vi "Autonomous Independent.vi"   [LabVIEW 2015]
doc: "This VI is called when autonomous begins, and will automatically be terminated when autonomous ends. You can carry out timed or sensor driven robot movement independently without needing to return to the caller."
uses:
  <vilib>/Rock Robotics/WPI/Relay/WPI_RelayValue.ctl
panel:
  # "Be sure to right-click and choose Data Operations>>Make Current Value default if you want to save the array values with the VI"
types:
  T1 = typedef "WPI_RelayDevRef.ctl" = cluster{"DevStatus":errorcluster, "Relay Channel":T2, "Relay Direction":T3}
  T2 = typedef "FPGA_DIORelayChannel.ctl" = enum8{"Relay 0", "Relay 1", "Relay 2", "Relay 3", "Invalid"}
  T3 = typedef "WPI_RelayDirection.ctl" = enum16{"Both directions", "Forward only", "Reverse only"}
  T4 = typedef "WPI_MotorControlDeviceRef.ctl" = cluster{"DeviceStatus":errorcluster, "Type":T5, "PWM":cluster{"PWM Channel":T6, "DeadBand":T7}, "CAN":cluster{"Device Number":u8, "Control Mode":T8, "Semaphore":T9, "Max Vout":dbl, "TalonSRX Control Mode":T10}, "Invert":bool}
  T5 = typedef "WPI_MotorControlType.ctl" = enum16{"PWM", "CAN", "CANTalonSRX"}
  T6 = typedef "FPGA_DIOPWMChannel.ctl" = enum8{"PWM 0", "PWM 1", "PWM 2", "PWM 3", "PWM 4", "PWM 5", "PWM 6", "PWM 7", "PWM 8", "PWM 9", "PWM MXP 0", "PWM MXP 1", "PWM MXP 2", "PWM MXP 3", "PWM MXP 4", "PWM MXP 5", "PWM MXP 6", "PWM MXP 7", "PWM MXP 8", "PWM MXP 9", "Invalid"}
  T7 = typedef "WPI_PWMDeadband.ctl" = cluster{"Name":string, "maxPositivePwm":i32, "minPositivePwm":i32, "centerPwm":i32, "maxNegativePwm":i32, "minNegativePwm":i32, "angularRange":u16}
  T8 = typedef "WPI_CANJaguar_ControlMode.ctl" = enum8{"Percent VBus", "Current", "Speed", "Position", "Voltage"}
  T9 = typedef "Semaphore RefNum" = refnum<k1>
  T10 = typedef "WPI_CANTalonSRX_APIControlMode.ctl" = enum8{"Percent VBus", "Speed", "Position", "Slave", "Unchanged / Invalid", "Voltage Compensation", "Current", "Motion Profile"}
  T11 = typedef "WPI_RelayValue.ctl" = enum16{"Off", "On", "Forward", "Reverse"}
  T12 = typedef "WPI_SwitchDevRef.ctl" = cluster{"DevStatus":errorcluster, "DIO Channel":T13, "CntIndex":T14, "Normally Closed":bool}
  T13 = typedef "FPGA_DIOChannel.ctl" = enum8{"DIO 0", "DIO 1", "DIO 2", "DIO 3", "DIO 4", "DIO 5", "DIO 6", "DIO 7", "DIO 8", "DIO 9", "DIO MXP 0", "DIO MXP 1", "DIO MXP 2", "DIO MXP 3", "DIO MXP 4", "DIO MXP 5", "DIO MXP 6", "DIO MXP 7", "DIO MXP 8", "DIO MXP 9", "DIO MXP 10", "DIO MXP 11", "DIO MXP 12", "DIO MXP 13", "DIO MXP 14", "DIO MXP 15", "Invalid"}
  T14 = typedef "FPGA_CounterCtrSystemIndex.ctl" = enum8{"Ctr 0", "Ctr 1", "Ctr 2", "Ctr 3", "Ctr 4", "Ctr 5", "Ctr 6", "Ctr 7", "Invalid"}
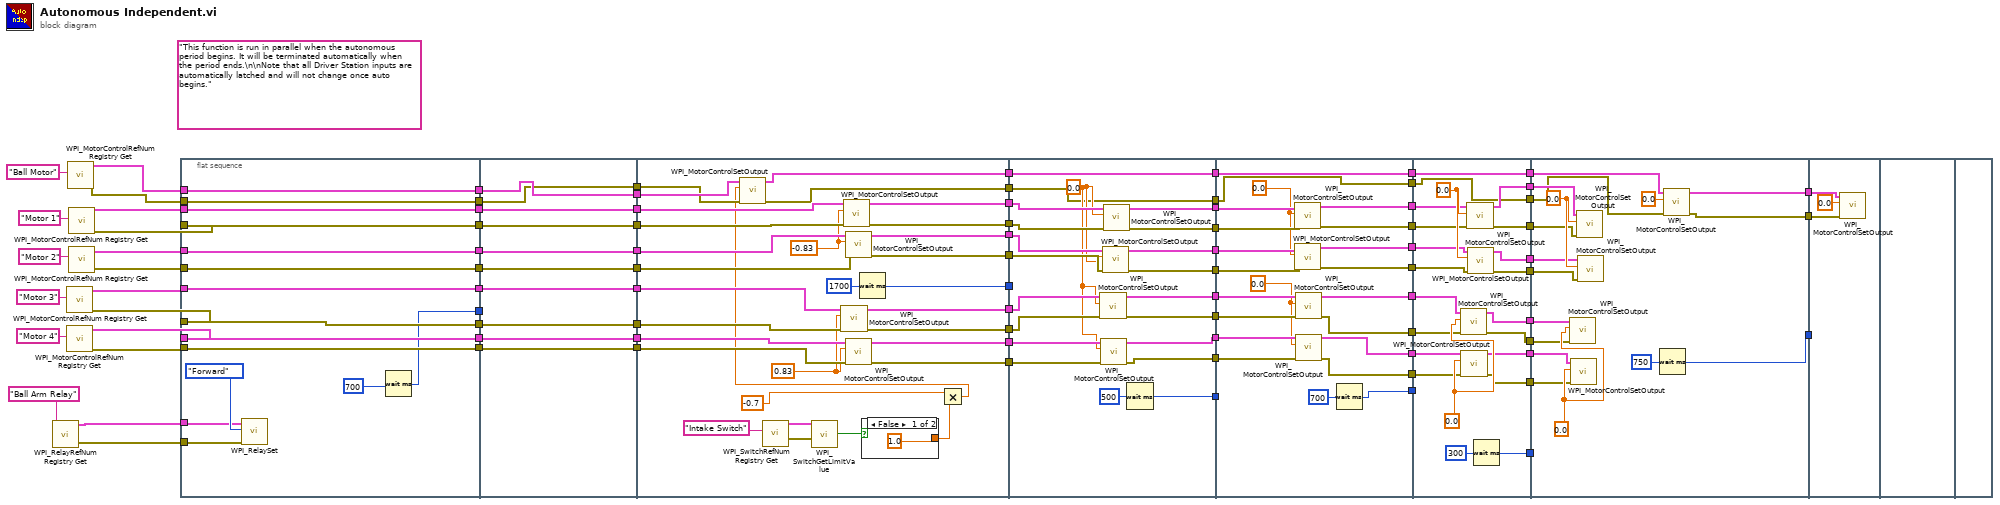
[diagram p0: block diagram]
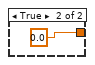
[diagram p2: hidden frame]
diagram:
  (unwired) "This function is run in parallel when the autonomous period begins. It will be terminated automatically when the period ends.\n\nNote that all Driver Station inputs are automatically latched and will not change once auto begins."
  n1 = call <vilib>:"WPI_RelayRefNum Registry Get.vi"("refnum name"="Ball Arm Relay") -> ("error out"=w72:errorcluster, "RelayDevRef"=w73:T1)  [unwired: 9 in]
  n2 = call <vilib>:"WPI_MotorControlRefNum Registry Get.vi"("refnum name"="Motor 3") -> ("error out"=w80:errorcluster, "MotorControlDevRef"=w79:T4)  [unwired: 9 in]
  n3 = call <vilib>:"WPI_MotorControlRefNum Registry Get.vi"("refnum name"="Motor 4") -> ("error out"=w81:errorcluster, "MotorControlDevRef"=w82:T4)  [unwired: 9 in]
  n4 = call <vilib>:"WPI_MotorControlRefNum Registry Get.vi"("refnum name"="Ball Motor") -> ("error out"=w51:errorcluster, "MotorControlDevRef"=w52:T4)  [unwired: 9 in]
  n5 = call <vilib>:"WPI_MotorControlRefNum Registry Get.vi"("refnum name"="Motor 1") -> ("error out"=w76:errorcluster, "MotorControlDevRef"=w75:T4)  [unwired: 9 in]
  n6 = call <vilib>:"WPI_MotorControlRefNum Registry Get.vi"("refnum name"="Motor 2") -> ("error out"=w78:errorcluster, "MotorControlDevRef"=w77:T4)  [unwired: 9 in]
  n7 = flat-sequence {
    tunnel: w75 -> [w94]
    tunnel: w76 -> [w95]
    tunnel: w77 -> [w96]
    tunnel: w78 -> [w97]
    tunnel: w79 -> [w98]
    tunnel: w80 -> [w99]
    tunnel: w81 -> [w100]
    tunnel: w82 -> [w101]
    tunnel: [w101] -> w70
    tunnel: [w100] -> w68
    tunnel: [w99] -> w66
    tunnel: [w98] -> w64
    tunnel: [w97] -> w62
    tunnel: [w96] -> w60
    tunnel: [w95] -> w58
    tunnel: [w94] -> w56
    tunnel: w73 -> [w92]
    tunnel: w72 -> [w91]
    tunnel: [w89] -> w54
    tunnel: [w88] -> w53
    tunnel: w52 -> [w88]
    tunnel: w51 -> [w87]
    tunnel: [w87] -> w50
    tunnel: w70 -> [w111]
    tunnel: [w111] -> w69
    tunnel: w68 -> [w110]
    tunnel: [w110] -> w67
    tunnel: w66 -> [w109]
    tunnel: [w109] -> w65
    tunnel: w64 -> [w108]
    tunnel: [w108] -> w63
    tunnel: w62 -> [w107]
    tunnel: [w107] -> w61
    tunnel: w60 -> [w106]
    tunnel: [w106] -> w59
    tunnel: w58 -> [w105]
    tunnel: [w105] -> w57
    tunnel: w56 -> [w104]
    tunnel: [w104] -> w55
    tunnel: w54 -> [_]
    tunnel: w53 -> [w103]
    tunnel: w50 -> [w102]
    tunnel: [w103] -> w49
    tunnel: [w102] -> w48
    tunnel: [w132] -> w47
    tunnel: [w131] -> w46
    tunnel: [w130] -> w45
    tunnel: [w129] -> w44
    tunnel: [w128] -> w43
    tunnel: [w127] -> w42
    tunnel: [w126] -> w41
    tunnel: [w125] -> w40
    tunnel: w69 -> [w142]
    tunnel: w67 -> [w141]
    tunnel: w65 -> [w140]
    tunnel: w63 -> [w139]
    tunnel: w61 -> [w138]
    tunnel: w59 -> [w137]
    tunnel: w57 -> [w136]
    tunnel: w55 -> [w135]
    tunnel: [w123] -> w39
    tunnel: w49 -> [w122]
    tunnel: w48 -> [w121]
    tunnel: [w113] -> w9
    tunnel: [w112] -> w6
    tunnel: w47 -> [w158]
    tunnel: w46 -> [w159]
    tunnel: w45 -> [w160]
    tunnel: w44 -> [w161]
    tunnel: w43 -> [w163]
    tunnel: w42 -> [w162]
    tunnel: w41 -> [w165]
    tunnel: w40 -> [w164]
    tunnel: w39 -> [_]
    tunnel: [w156] -> w38
    tunnel: [w155] -> w37
    tunnel: [w154] -> w36
    tunnel: [w153] -> w35
    tunnel: [w152] -> w34
    tunnel: [w151] -> w33
    tunnel: [w150] -> w32
    tunnel: [w149] -> w31
    tunnel: [w148] -> w30
    tunnel: [w146] -> w10
    tunnel: w9 -> [w146]
    tunnel: [w145] -> w7
    tunnel: w6 -> [w145]
    tunnel: w38 -> [w187]
    tunnel: w37 -> [w186]
    tunnel: w36 -> [w185]
    tunnel: w35 -> [w184]
    tunnel: w34 -> [w183]
    tunnel: w33 -> [w182]
    tunnel: w32 -> [w181]
    tunnel: w31 -> [w180]
    tunnel: [w178] -> w29
    tunnel: w30 -> [_]
    tunnel: [w176] -> w28
    tunnel: [w175] -> w27
    tunnel: [w174] -> w26
    tunnel: [w173] -> w25
    tunnel: [w172] -> w24
    tunnel: [w171] -> w23
    tunnel: [w170] -> w22
    tunnel: [w169] -> w21
    tunnel: [w168] -> w11
    tunnel: w10 -> [w168]
    tunnel: [w167] -> w8
    tunnel: w7 -> [w167]
    tunnel: w29 -> [_]
    tunnel: w28 -> [w207]
    tunnel: w27 -> [w206]
    tunnel: w26 -> [w205]
    tunnel: w25 -> [w204]
    tunnel: w24 -> [w203]
    tunnel: w23 -> [w202]
    tunnel: w22 -> [w201]
    tunnel: w21 -> [w200]
    tunnel: [w199] -> w20
    tunnel: [w197] -> w19
    tunnel: [w196] -> w18
    tunnel: [w195] -> w17
    tunnel: [w194] -> w16
    tunnel: [w193] -> w15
    tunnel: [w192] -> w14
    tunnel: [w191] -> w13
    tunnel: [w190] -> w12
    tunnel: w11 -> [w189]
    tunnel: w8 -> [w188]
    tunnel: [w189] -> w5
    tunnel: [w188] -> w4
    tunnel: w20 -> [_]
    tunnel: w19 -> [w224]
    tunnel: w18 -> [w223]
    tunnel: w17 -> [w222]
    tunnel: w16 -> [w221]
    tunnel: w15 -> [w220]
    tunnel: w14 -> [w219]
    tunnel: w13 -> [w218]
    tunnel: w12 -> [w217]
    tunnel: w5 -> [w216]
    tunnel: w4 -> [w215]
    tunnel: [w212] -> w3
    tunnel: [w211] -> w2
    tunnel: [w210] -> w1
    tunnel: w3 -> [_]
    tunnel: w2 -> [w229]
    tunnel: w1 -> [w228]
    frame #0 {
      n8 = call <vilib>:"WPI_RelaySet.vi"("error in (no error)"=w91, "RelayValue"=WPI_RelayValue."Forward", "RelayDevRef"=w92) -> ()  [unwired: 7 in, 2 out]
      n9 = Wait (ms)(milliseconds to wait=u32 700) -> (millisecond timer value=w89:u32)
    }
    frame #1 {
    }
    frame #2 {
      w133 = 0.83
      w134 = -0.83
      n10 = call <vilib>:"WPI_SwitchRefNum Registry Get.vi"("refnum name"="Intake Switch") -> ("error out"=w119:errorcluster, "SwitchDevRef"=w120:T12)  [unwired: 9 in]
      n11 = call <vilib>:"WPI_SwitchGetLimitValue.vi"("error in (no error)"=w119, "SwitchDevRef"=w120) -> ("Switch Pressed"=w114:bool)  [unwired: 7 in, 2 out]
      n12 = call <vilib>:"WPI_MotorControlSetOutput.vi"("error in (no error)"=w140, "Output"=w133, "MotorControlDevRef"=w139) -> ("error out"=w127:errorcluster, "MotorControlDevRef"=w128:T4)  [unwired: 6 in, 1 out]
      n13 = call <vilib>:"WPI_MotorControlSetOutput.vi"("error in (no error)"=w136, "Output"=w134, "MotorControlDevRef"=w135) -> ("error out"=w131:errorcluster, "MotorControlDevRef"=w132:T4)  [unwired: 6 in, 1 out]
      n14 = call <vilib>:"WPI_MotorControlSetOutput.vi"("error in (no error)"=w138, "Output"=w134, "MotorControlDevRef"=w137) -> ("error out"=w129:errorcluster, "MotorControlDevRef"=w130:T4)  [unwired: 6 in, 1 out]
      n15 = call <vilib>:"WPI_MotorControlSetOutput.vi"("error in (no error)"=w141, "Output"=w133, "MotorControlDevRef"=w142) -> ("error out"=w125:errorcluster, "MotorControlDevRef"=w126:T4)  [unwired: 6 in, 1 out]
      n16 = Wait (ms)(milliseconds to wait=u32 1700) -> (millisecond timer value=w123:u32)
      n17 = case shown="False" w114 {
        tunnel: [1.0 0.0] -> w117
        frame False {
        }
        frame True {
        }
      }
      n18 = Multiply(x=-0.7 ("Output"), y=w117) -> (x*y=w115:dbl)
      n19 = call <vilib>:"WPI_MotorControlSetOutput.vi"("error in (no error)"=w121, "Output"=w115, "MotorControlDevRef"=w122) -> ("error out"=w112:errorcluster, "MotorControlDevRef"=w113:T4)  [unwired: 6 in, 1 out]
    }
    frame #3 {
      w157 = 0.0 ("Output")
      n20 = call <vilib>:"WPI_MotorControlSetOutput.vi"("error in (no error)"=w162, "Output"=w157, "MotorControlDevRef"=w163) -> ("error out"=w149:errorcluster, "MotorControlDevRef"=w150:T4)  [unwired: 6 in, 1 out]
      n21 = call <vilib>:"WPI_MotorControlSetOutput.vi"("error in (no error)"=w164, "Output"=w157, "MotorControlDevRef"=w165) -> ("error out"=w151:errorcluster, "MotorControlDevRef"=w152:T4)  [unwired: 6 in, 1 out]
      n22 = call <vilib>:"WPI_MotorControlSetOutput.vi"("error in (no error)"=w161, "Output"=w157, "MotorControlDevRef"=w160) -> ("error out"=w153:errorcluster, "MotorControlDevRef"=w154:T4)  [unwired: 6 in, 1 out]
      n23 = call <vilib>:"WPI_MotorControlSetOutput.vi"("error in (no error)"=w159, "Output"=w157, "MotorControlDevRef"=w158) -> ("error out"=w155:errorcluster, "MotorControlDevRef"=w156:T4)  [unwired: 6 in, 1 out]
      n24 = Wait (ms)(milliseconds to wait=u32 500) -> (millisecond timer value=w148:u32)
    }
    frame #4 {
      w166 = 0.0 ("Output")
      w179 = 0.0 ("Output")
      n25 = call <vilib>:"WPI_MotorControlSetOutput.vi"("error in (no error)"=w186, "Output"=w179, "MotorControlDevRef"=w187) -> ("error out"=w175:errorcluster, "MotorControlDevRef"=w176:T4)  [unwired: 6 in, 1 out]
      n26 = call <vilib>:"WPI_MotorControlSetOutput.vi"("error in (no error)"=w184, "Output"=w179, "MotorControlDevRef"=w185) -> ("error out"=w173:errorcluster, "MotorControlDevRef"=w174:T4)  [unwired: 6 in, 1 out]
      n27 = call <vilib>:"WPI_MotorControlSetOutput.vi"("error in (no error)"=w180, "Output"=w166, "MotorControlDevRef"=w181) -> ("error out"=w171:errorcluster, "MotorControlDevRef"=w172:T4)  [unwired: 6 in, 1 out]
      n28 = call <vilib>:"WPI_MotorControlSetOutput.vi"("error in (no error)"=w182, "Output"=w166, "MotorControlDevRef"=w183) -> ("error out"=w169:errorcluster, "MotorControlDevRef"=w170:T4)  [unwired: 6 in, 1 out]
      n29 = Wait (ms)(milliseconds to wait=u32 700) -> (millisecond timer value=w178:u32)
    }
    frame #5 {
      w209 = 0.0 ("Output")
      w208 = 0.0 ("Output")
      n30 = call <vilib>:"WPI_MotorControlSetOutput.vi"("error in (no error)"=w202, "Output"=w209, "MotorControlDevRef"=w203) -> ("error out"=w192:errorcluster, "MotorControlDevRef"=w193:T4)  [unwired: 6 in, 1 out]
      n31 = call <vilib>:"WPI_MotorControlSetOutput.vi"("error in (no error)"=w200, "Output"=w209, "MotorControlDevRef"=w201) -> ("error out"=w190:errorcluster, "MotorControlDevRef"=w191:T4)  [unwired: 6 in, 1 out]
      n32 = call <vilib>:"WPI_MotorControlSetOutput.vi"("error in (no error)"=w206, "Output"=w208, "MotorControlDevRef"=w207) -> ("error out"=w196:errorcluster, "MotorControlDevRef"=w197:T4)  [unwired: 6 in, 1 out]
      n33 = call <vilib>:"WPI_MotorControlSetOutput.vi"("error in (no error)"=w204, "Output"=w208, "MotorControlDevRef"=w205) -> ("error out"=w194:errorcluster, "MotorControlDevRef"=w195:T4)  [unwired: 6 in, 1 out]
      n34 = Wait (ms)(milliseconds to wait=u32 300) -> (millisecond timer value=w199:u32)
    }
    frame #6 {
      w225 = 0.0 ("Output")
      w226 = 0.0 ("Output")
      n35 = call <vilib>:"WPI_MotorControlSetOutput.vi"("error in (no error)"=w219, "Output"=w225, "MotorControlDevRef"=w220) -> ()  [unwired: 6 in, 3 out]
      n36 = call <vilib>:"WPI_MotorControlSetOutput.vi"("error in (no error)"=w217, "Output"=w225, "MotorControlDevRef"=w218) -> ()  [unwired: 6 in, 3 out]
      n37 = call <vilib>:"WPI_MotorControlSetOutput.vi"("error in (no error)"=w223, "Output"=w226, "MotorControlDevRef"=w224) -> ()  [unwired: 6 in, 3 out]
      n38 = call <vilib>:"WPI_MotorControlSetOutput.vi"("error in (no error)"=w221, "Output"=w226, "MotorControlDevRef"=w222) -> ()  [unwired: 6 in, 3 out]
      n39 = Wait (ms)(milliseconds to wait=u32 750) -> (millisecond timer value=w212:u32)
      n40 = call <vilib>:"WPI_MotorControlSetOutput.vi"("error in (no error)"=w215, "Output"=0.0, "MotorControlDevRef"=w216) -> ("error out"=w210:errorcluster, "MotorControlDevRef"=w211:T4)  [unwired: 6 in, 1 out]
    }
    frame #7 {
      n41 = call <vilib>:"WPI_MotorControlSetOutput.vi"("error in (no error)"=w228, "Output"=0.0, "MotorControlDevRef"=w229) -> ()  [unwired: 6 in, 3 out]
    }
    frame #8 {
    }
    frame #9 {
    }
  }
